vi "Write PowerSV.vi"(8 "error in (no error)":errorcluster, 10 "PowerSV":refnum<k21>, 11 "FlipMir in":refnum<class "FlipMir.lvclass">) -> (0 "error out":errorcluster, 3 "FlipMir out":refnum<class "FlipMir.lvclass">)   [LabVIEW 2016, in "FlipMir.lvclass"]
uses:
  FlipMir.lvclass
  FlipMir.lvclass/FlipMir.ctl
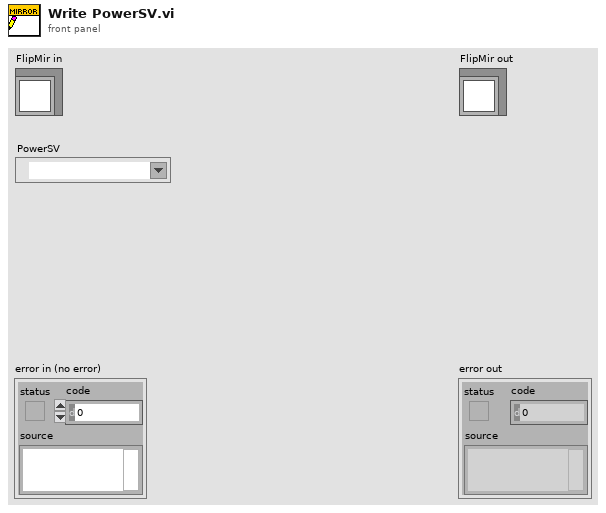
[diagram p1: front panel]
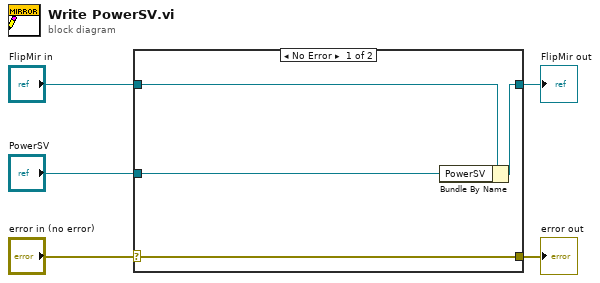
[diagram p0: block diagram]
diagram:
  n1 = case shown="No Error" "error in (no error)" {
    selector: "error in (no error)" -> [w9 w10]
    tunnel: [w9 w10] -> w4
    tunnel: [w7 w11] -> w2
    tunnel: "FlipMir in" -> [w8 w11]
    tunnel: "PowerSV" -> [w6 _]
    frame No Error {
      n2 = Bundle By Name(cluster=w8, "PowerSV"=w6) -> (w7:refnum<class "FlipMir.lvclass">)
    }
    frame Error {
    }
  }
  "error out" <- w4
  "FlipMir out" <- w2
